vi "Test OAuth2.vi"() -> ()   [LabVIEW 2020]
uses:
  OAuth2/Client/Client.lvclass
  OAuth2/Request/Request.lvclass
  OAuth2/OAuth2/OAuth2.lvclass
  OAuth2/Async Authorization/Async Authorization.lvclass
  OAuth2/Authorization/Authorization.lvclass
  OAuth2/Async Auth State.ctl
  OAuth2/OAuth2.lvlib
  OAuth2/Expiry.ctl
panel:
  out "Refresh Expiry":T1
  out "Expiry":T1
  out "error out":errorcluster
  out "State":T2
  in  "Scopes":string[](array[string])
  in  "Redirect URL":string
  in  "Token URL":string
  in  "Auth URL":string
  in  "Client Secret":string
  in  "Client ID":string
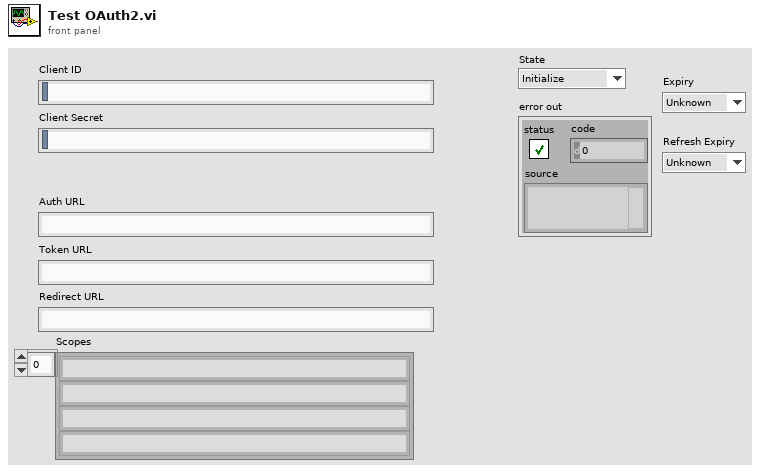
[diagram p1: front panel]
types:
  T1 = typedef "OAuth2.lvlib/Expiry.ctl" = enum16{"Unknown", "Expired", "Good"}
  T2 = typedef "OAuth2.lvlib/Async Auth State.ctl" = enum16{"Initialize", "Request", "WaitAuth", "GetToken", "RefreshToken", "Complete", "Failed"}
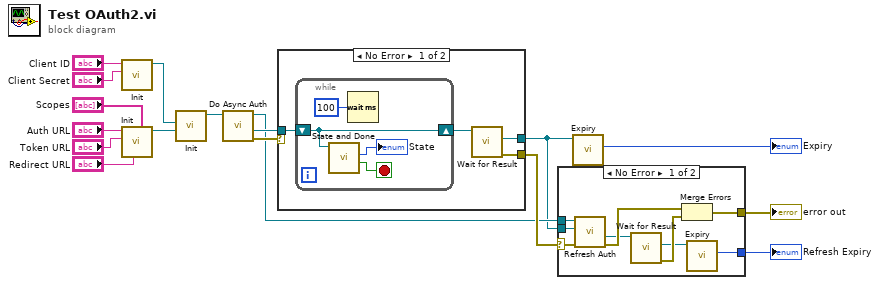
[diagram p0: block diagram]
diagram:
  n1 = call "Init.vi"("Secret"="Client Secret", "ID"="Client ID") -> ("Client out"=w9:refnum<class "Client.lvclass">)  [unwired: 9 in]
  n2 = call "Init.vi"("Required Scope(s)"="Scopes", "Redirect URL (http://localhost)"="Redirect URL", "Token URL"="Token URL", "Auth URL"="Auth URL") -> ("Request out"=w10:refnum<class "Request.lvclass">)  [unwired: 7 in]
  n3 = call "Init.vi"("Request"=w10, "Client"=w9) -> ("OAuth2"=w13:refnum<class "OAuth2.lvclass">)  [unwired: 9 in]
  n4 = call "Do Async Auth.vi"("OAuth2 in"=w13) -> ("error out"=w12:errorcluster, "Async Authentication"=w3:refnum<class "Async Authorization.lvclass">, "OAuth2 out"=w2:refnum<class "OAuth2.lvclass">)  [unwired: 8 in]
  n5 = case shown="No Error" w12 {
    selector: w12 -> [_ w26]
    tunnel: w3 -> [w21 _]
    tunnel: [w19 w26] -> w17
    tunnel: [w18 _] -> w1
    frame No Error {
      n6 = while {
        shift-right: [w23] -> w20
        shift-left: w21 -> [w23]
        stop <- w25 stop-if-true
        n7 = call "State and Done.vi"("Async Authorization in"=w23) -> ("Done?"=w25:bool, "State"=→"State":T2)  [unwired: 9 in]
        n8 = Wait (ms)(milliseconds to wait=u32 100) -> ()  [unwired: 1 out]
      }
      n9 = call "Wait for Result.vi"("Async Authorization in"=w20) -> ("error out"=w19:errorcluster, "Authorization"=w18:refnum<class "Authorization.lvclass">)  [unwired: 8 in, 1 out]
    }
    frame Error {
    }
  }
  n10 = case shown="No Error" w17 {
    selector: w17 -> [w34 w36]
    tunnel: w2 -> [w33 _]
    tunnel: [w30 w36] -> w5
    tunnel: w1 -> [w29 _]
    tunnel: [w27 _] -> w4
    frame No Error {
      n11 = call "Refresh Auth.vi"("error in (no error)"=w34, "Authorization in"=w29, "OAuth2 in"=w33) -> ("error out"=w35:errorcluster, "Async Authentication"=w32:refnum<class "Async Authorization.lvclass">)  [unwired: 6 in, 1 out]
      n12 = call "Wait for Result.vi"("Async Authorization in"=w32) -> ("error out"=w31:errorcluster, "Authorization"=w28:refnum<class "Authorization.lvclass">)  [unwired: 8 in, 1 out]
      n13 = Merge Errors(w35, w31) -> (w30:errorcluster)
      n14 = call "Expiry.vi"("Authorization in"=w28) -> ("Expiry"=w27:T1)  [unwired: 10 in]
    }
    frame Error {
    }
  }
  "error out" <- w5
  "Refresh Expiry" <- w4
  n15 = call "Expiry.vi"("Authorization in"=w1) -> ("Expiry"=→"Expiry":T1)  [unwired: 10 in]
